vi "Actor Core.vi"(8 "error in":errorcluster, 11 "SensorViewDetailed in":refnum<class "SensorViewDetailed.lvclass">) -> (0 "error out":errorcluster, 3 "Actor out":refnum<class "Actor.lvclass">)   [LabVIEW 2012, in "Sensor Definition.lvlib" / "SensorViewDetailed.lvclass"]
doc: "(<B>Filename</B>: Actor Framework.lvlib:Actor.lvclass:Actor Core.vi)\n\nReceives messages to the actor, reacts to them, and initiates any error handling that may shut the actor down.\n\nDescendant classes may override this VI to append parallel tasks for the actor to complete while it handles messages. Overrides use the Call Parent Method node."
uses:
  SensorViewDetailed.lvclass
  <vilib>/ActorFramework/Actor/Actor.lvclass
  Controls/String XControl/String XControl.xctl
  SensorView.lvclass
  <vilib>/ActorFramework/Actor/Actor.lvclass/Actor.ctl
  <vilib>/ActorFramework/Message Enqueuer/Message Enqueuer.lvclass/Message Enqueuer.ctl
  Win8uiFramework/ViewableActor.lvclass/ViewableActor.ctl
  SensorView.lvclass/SensorView.ctl
  Sensor Messages/Request Detach Msg/Request Detach Msg.lvclass/Request Detach Msg.ctl
  SensorInfo.lvclass/SensorInfo.ctl
  Double Scalar SensorData.lvclass
  SensorInfo/Read Description.vi
  SensorInfo/Read Name.vi
  Win8uiFramework/Read Stop Event.vi
  SensorView/Read SensorInfo Changed Event.vi
  SensorView/Read SensorData Changed Event.vi
  <vilib>/ActorFramework/Message Enqueuer/Init from Existing Queue.vi
  <vilib>/ActorFramework/Message Enqueuer/Enqueue.vi
  <vilib>/ActorFramework/Message Priority Queue/Priority Enqueue.vi
  <vilib>/ActorFramework/Message Enqueuer/Message Enqueuer.lvclass
  SensorInfo.lvclass
  SensorData.lvclass
  <vilib>/ActorFramework/Stop Msg/Stop Msg.lvclass
  Sensor Messages/Request Display Charm Msg/Request Display Charm Msg.lvclass
  Sensor Messages/Request Detach Msg/Request Detach Msg.lvclass
  Sensor Messages/Shutdown Sensor Msg/Shutdown Sensor Msg.lvclass
  Win8uiFramework/ViewableActor.lvclass
  Win8uiFramework/Win8uiFramework.lvlib
panel:
  out "Title":string(xcontrol)
  out "Description":string="Application Title"
  out "Waveform Chart":dbl(graph)
  in  "Delete":bool
  in  "Open in New Window Button":bool
  in  "Settings":bool
  in  "Back Button":bool
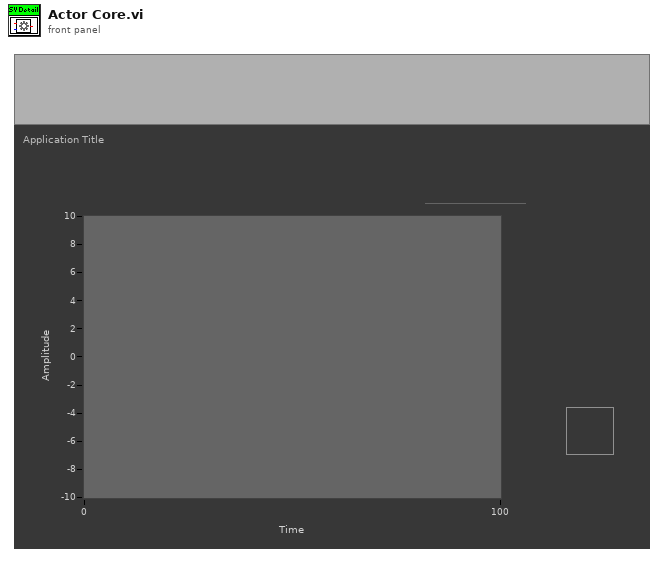
[diagram p1: front panel]
types:
  T1 = cluster{"horizontal":enum16{"left", "center", "right"}, "vertical":enum16{"top", "center", "bottom"}}
  T2 = cluster{"Font Name:":string, "Size":i16, "Strikeout?":bool, "Italic?":bool, "Underline?":bool, "Outline?":bool, "Shadow?":bool, "Bold?":bool}
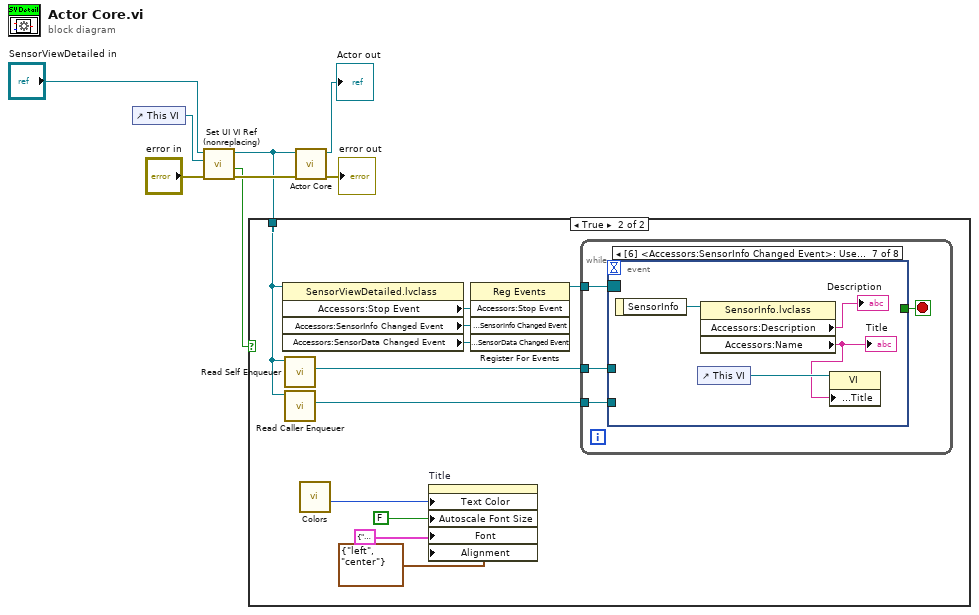
[diagram p0: block diagram]
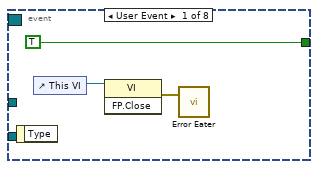
[diagram p3: hidden frame]
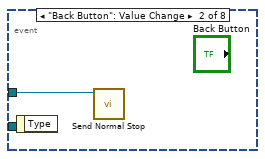
[diagram p4: hidden frame]
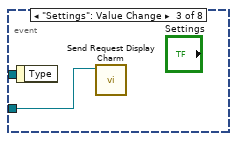
[diagram p5: hidden frame]
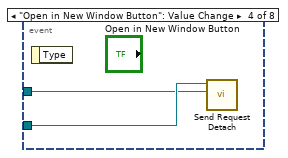
[diagram p6: hidden frame]
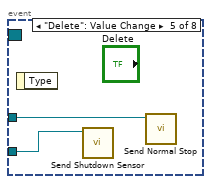
[diagram p7: hidden frame]
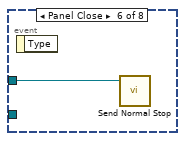
[diagram p8: hidden frame]
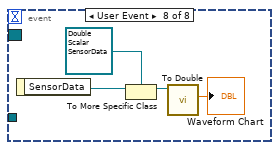
[diagram p9: hidden frame]
diagram:
  n1 = control-ref of="This VI"() -> (w6:refnum<vi>)
  n2 = call "Set UI VI Ref (nonreplacing).vi"("error in (no error)"="error in", "UI VI Ref"=w6, "ViewableActor in"="SensorViewDetailed in") -> ("error out"=w4:errorcluster, "Top Level UI?"=w2:bool, "ViewableActor out"=w3:refnum<class "SensorViewDetailed.lvclass">)  [unwired: 6 in]
  n3 = case shown="True" w2 {
    tunnel: w3 -> [_ w14]
    frame False {
    }
    frame True {
      n4 = property class="SensorViewDetailed.lvclass"(reference=w14) -> ("Accessors:Stop Event"=w19:refnum<user-event>, "Accessors:SensorInfo Changed Event"=w18:refnum<user-event>, "Accessors:SensorData Changed Event"=w16:refnum<user-event>)  [unwired: 1 in, 2 out]
      n5 = call <vilib>:"Read Self Enqueuer.vi"("Actor"=w14) -> ("Self Enqueuer"=w15:refnum<class "Message Enqueuer.lvclass">)  [unwired: 10 in]
      n6 = call <vilib>:"Read Caller Enqueuer.vi"("Actor"=w14) -> ("Caller Enqueuer"=w13:refnum<class "Message Enqueuer.lvclass">)  [unwired: 10 in]
      n7 = call "Colors.vi"() -> ("Text Color"=w12:u32)  [unwired: 8 in, 3 out]
      n8 = property on="Title" class="String XControl (strict)"("Text Color"=w12, "Autoscale Font Size"=FALSE, "Font"=T2 {"Font Name:"="Segoe UI", "Size"=48, "Strikeout?"=FALSE, "Italic?"=FALSE, "Underline?"=FALSE, "Outline?"=FALSE, "Shadow?"=FALSE, "Bold?"=FALSE}, "Alignment"=T1 {"horizontal"=enum."left", "vertical"=enum."center"}) -> ()  [unwired: 2 in, 2 out]
      n9 = register-events(w19, w18, w16) -> (reference out=w17:refnum<event-registration>)  [unwired: 2 in, 1 out]
      n10 = while {
        tunnel: w17 -> [w23]
        tunnel: w15 -> [w21]
        tunnel: w13 -> [w20]
        stop <- w22 stop-if-true
        n11 = event shown="[6] <Accessors:SensorInfo Changed Event>: User Event" {
          selector: w23 -> [_ _ _ _ _ _ _ _]
          dyn-events: _ -> [_ _ _ _ _ _ _ _]
          timeout: _ -> [_ _ _ _ _ _ _ _]
          tunnel: [TRUE _ _ _ _ _ _ _] -> w22
          tunnel: w21 -> [_ w27 _ w29 w32 w33 _ _]
          tunnel: w20 -> [_ _ w28 w30 w31 _ _ _]
          event User Event {
            n12 = event-data() -> ()  [unwired: 1 in, 1 out]
            n13 = control-ref of="This VI"() -> (w24:refnum<vi>)
            n14 = invoke class="VI" method="FP.Close"(reference=w24) -> (error out=w25:errorcluster)  [unwired: 2 in, 2 out]
            n15 = call "Error Eater.vi"("error in (no error)"=w25) -> ()  [unwired: 2 in]
          }
          event "Back Button": Value Change {
            n16 = event-data() -> ()  [unwired: 1 in, 1 out]
            n17 = call <vilib>:"Send Normal Stop.vi"("Message Enqueuer"=w27) -> ()  [unwired: 10 in, 1 out]
          }
          event "Settings": Value Change {
            n18 = event-data() -> ()  [unwired: 1 in, 1 out]
            n19 = call "Send Request Display Charm.vi"("Message Enqueuer"=w28) -> ()  [unwired: 9 in, 2 out]
          }
          event "Open in New Window Button": Value Change {
            n20 = event-data() -> ()  [unwired: 1 in, 1 out]
            n21 = call "Send Request Detach.vi"("SensorView Enqueuer"=w29, "Message Enqueuer"=w30) -> ()  [unwired: 8 in, 2 out]
          }
          event "Delete": Value Change {
            n22 = event-data() -> ()  [unwired: 1 in, 1 out]
            n23 = call "Send Shutdown Sensor.vi"("Message Enqueuer"=w31) -> ()  [unwired: 9 in, 2 out]
            n24 = call <vilib>:"Send Normal Stop.vi"("Message Enqueuer"=w32) -> ()  [unwired: 10 in, 1 out]
          }
          event Panel Close {
            n25 = event-data() -> ()  [unwired: 1 in, 1 out]
            n26 = call <vilib>:"Send Normal Stop.vi"("Message Enqueuer"=w33) -> ()  [unwired: 10 in, 1 out]
          }
          event User Event {
            n27 = event-data() -> ("SensorInfo"=w37:refnum<class "SensorInfo.lvclass">)  [unwired: 1 in]
            n28 = control-ref of="This VI"() -> (w36:refnum<vi>)
            n29 = property class="SensorInfo.lvclass"(reference=w37) -> ("Accessors:Description"=→"Description":string, "Accessors:Name"=w35:string)  [unwired: 1 in, 2 out]
            "Title" <- w35
            n30 = property class="VI"(reference=w36, "Front Panel.Title"=w35) -> ()  [unwired: 1 in, 2 out]
          }
          event User Event {
            n31 = event-data() -> ("SensorData"=w41:refnum<class "SensorData.lvclass">)  [unwired: 1 in]
            n32 = To More Specific Class(target class=refnum<class "Double Scalar SensorData.lvclass"> refnum ("Sensor Definition.lvlib:Double Scalar SensorData.lvclass"), reference=w41) -> (specific class reference=w40:refnum<class "Double Scalar SensorData.lvclass">)  [unwired: 1 in, 1 out]
            n33 = call-dynamic "To Double.vi"("Double Scalar SensorData in"=w40) -> ("Value"=→"Waveform Chart":dbl)  [unwired: 8 in, 2 out]
          }
        }
      }
    }
  }
  n34 = call-parent "Actor Core.vi"("error in"=w4, "Actor in"=w3) -> ("error out"=→"error out":errorcluster, "Actor out"=→"Actor out":refnum<class "Actor.lvclass">)  [unwired: 8 in]
